vi "单个流程写入.vi"(7 "添加的路径":path, 8 "error in (no error)":errorcluster caption="错误输入（无错误）", 9 "量程":enum16{"低量程", "高量程"}(ring), 10 "测量模式":enum16{"水样测量", "零点核查", "跨度核查", "标样核查", "加标回收"}(ring), 11 "测量参数":enum16{"总磷", "总氮", "氨氮"}(ring)) -> (0 "error out":errorcluster caption="错误输出")   [LabVIEW 2016, in "斯坦道总磷.lvlib"]
panel:
  out "数组 2":u16[][](array[numeric])
  out "大小":i32
  out "交织的数组":u16[](array[numeric]) format="%04x"
  out "数值":i32
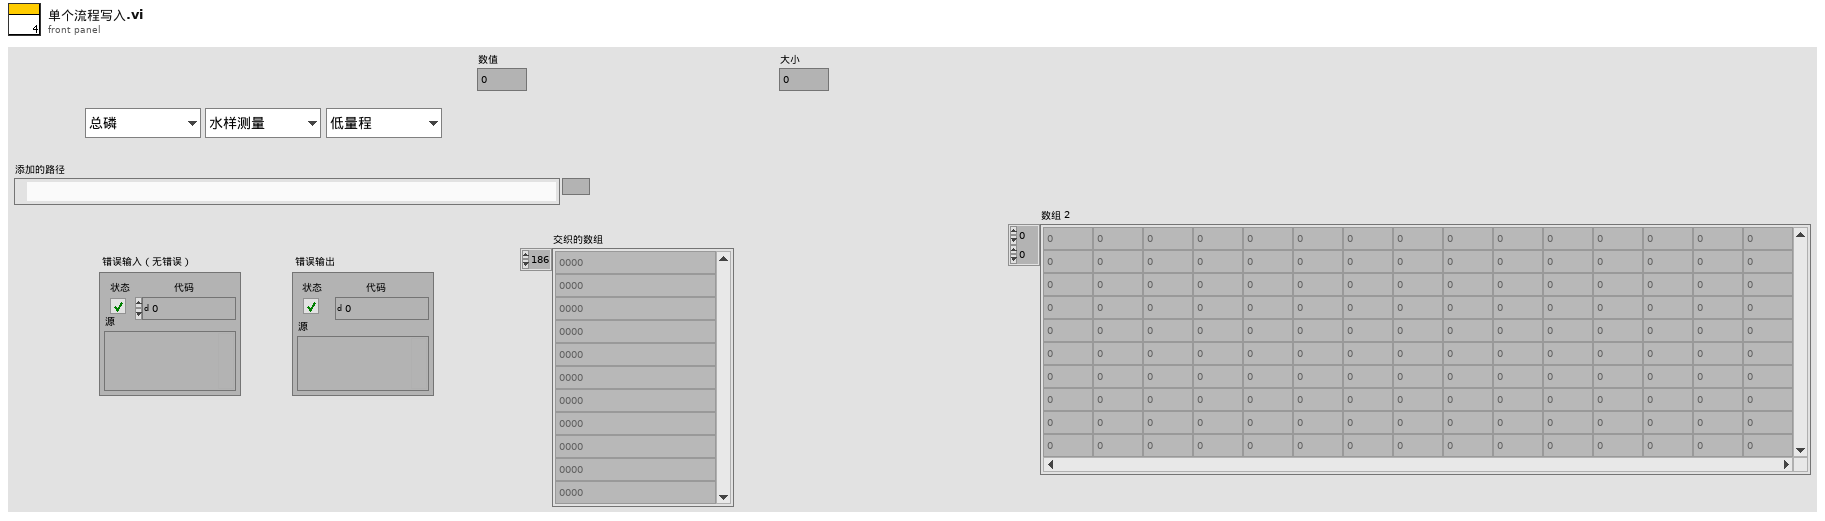
[diagram p1: front panel]
types:
  T1 = cluster{"站号":u16, "starting address":u16, "starting address":u16}
  T2 = cluster{"port":u32, "dac":u8, "adc":u8, "time":u16, "步骤名":string}[]
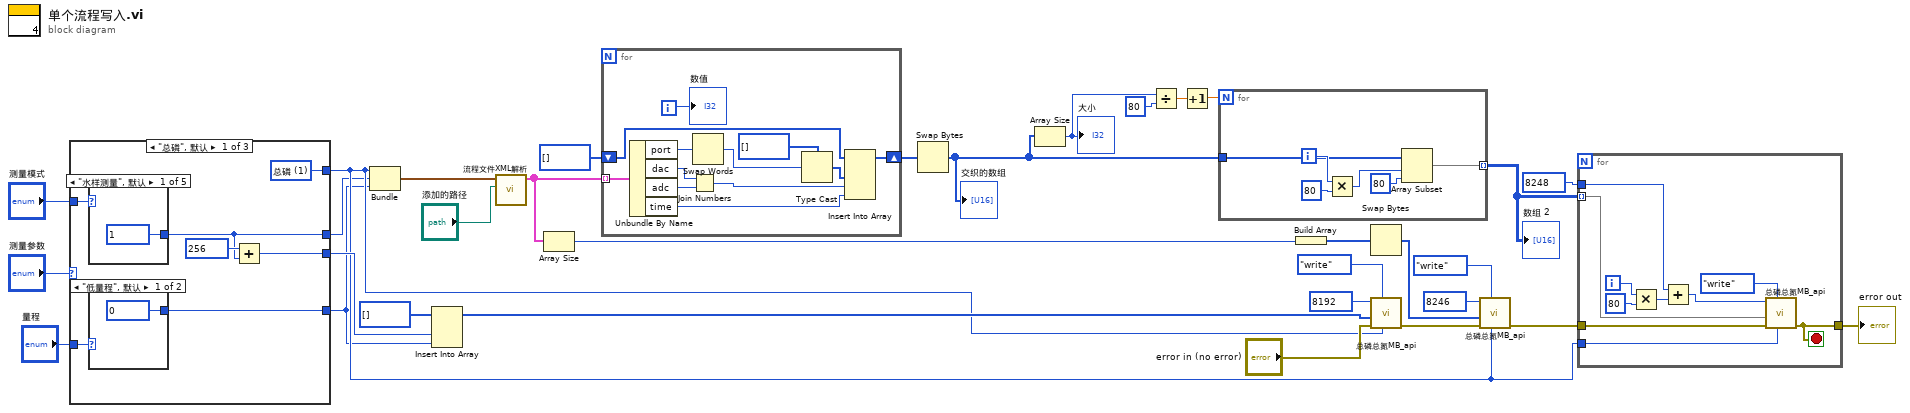
[diagram p0: block diagram]
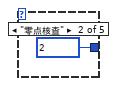
[diagram p2: hidden frame]
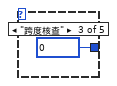
[diagram p3: hidden frame]
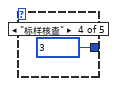
[diagram p4: hidden frame]
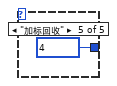
[diagram p5: hidden frame]
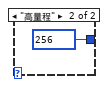
[diagram p6: hidden frame]
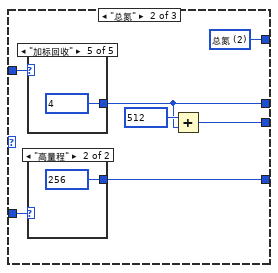
[diagram p7: hidden frame]
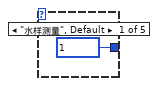
[diagram p8: hidden frame]
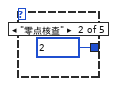
[diagram p9: hidden frame]
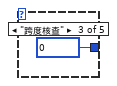
[diagram p10: hidden frame]
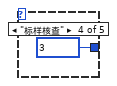
[diagram p11: hidden frame]
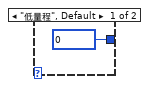
[diagram p12: hidden frame]
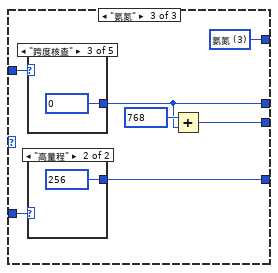
[diagram p13: hidden frame]
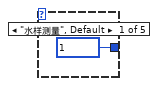
[diagram p14: hidden frame]
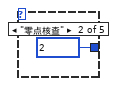
[diagram p15: hidden frame]
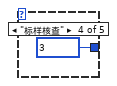
[diagram p16: hidden frame]
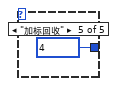
[diagram p17: hidden frame]
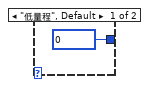
[diagram p18: hidden frame]
diagram:
  n1 = case shown="\"总磷\", 默认" "测量参数" {
    tunnel: "测量模式" -> [w38 w51 w65]
    tunnel: "量程" -> [w39 w52 w66]
    tunnel: [w34 w53 w67] -> w18
    tunnel: [w35 w48 w62] -> w28
    tunnel: [w37 w50 w64] -> w15
    tunnel: [w33 w47 w61] -> w16
    frame "总磷", Default {
      w34 = u16 1 items=["总磷"=1, "总氮"=2, "氨氮"=3] ("站号")
      n2 = case shown="\"水样测量\", 默认" w38 {
        tunnel: [u16 1 ("starting address") u16 2 ("starting address") u16 0 ("starting address") u16 3 ("starting address") u16 4 ("starting address")] -> w33
        frame "水样测量", Default {
        }
        frame "零点核查" {
        }
        frame "跨度核查" {
        }
        frame "标样核查" {
        }
        frame "加标回收" {
        }
      }
      n3 = case shown="\"低量程\", 默认" w39 {
        tunnel: [u16 0 ("starting address") u16 256 ("starting address")] -> w37
        frame "低量程", Default {
        }
        frame "高量程" {
        }
      }
      n4 = Add(x=u16 256 ("starting address"), y=w33) -> (x+y=w35:u16)
    }
    frame "总氮" {
      w53 = u16 2 items=["总磷"=1, "总氮"=2, "氨氮"=3] ("站号")
      n5 = case shown="\"加标回收\"" w51 {
        tunnel: [u16 1 ("starting address") u16 2 ("starting address") u16 0 ("starting address") u16 3 ("starting address") u16 4 ("starting address")] -> w47
        frame "水样测量", Default {
        }
        frame "零点核查" {
        }
        frame "跨度核查" {
        }
        frame "标样核查" {
        }
        frame "加标回收" {
        }
      }
      n6 = case shown="\"高量程\"" w52 {
        tunnel: [u16 0 ("starting address") u16 256 ("starting address")] -> w50
        frame "低量程", Default {
        }
        frame "高量程" {
        }
      }
      n7 = Add(x=u16 512 ("starting address"), y=w47) -> (x+y=w48:u16)
    }
    frame "氨氮" {
      w67 = u16 3 items=["总磷"=1, "总氮"=2, "氨氮"=3] ("站号")
      n8 = case shown="\"跨度核查\"" w65 {
        tunnel: [u16 1 ("starting address") u16 2 ("starting address") u16 0 ("starting address") u16 3 ("starting address") u16 4 ("starting address")] -> w61
        frame "水样测量", Default {
        }
        frame "零点核查" {
        }
        frame "跨度核查" {
        }
        frame "标样核查" {
        }
        frame "加标回收" {
        }
      }
      n9 = case shown="\"高量程\"" w66 {
        tunnel: [u16 0 ("starting address") u16 256 ("starting address")] -> w64
        frame "低量程", Default {
        }
        frame "高量程" {
        }
      }
      n10 = Add(x=u16 768 ("starting address"), y=w61) -> (x+y=w62:u16)
    }
  }
  n11 = Bundle("站号"=w18, "starting address"=w16, "starting address"=w15) -> (w14:T1)  [unwired: 1 in]
  n12 = Insert Into Array(array=u16[] [] ("数组"), new element #1=w28, new element #2=w15) -> (w22:u16[])  [unwired: 1 in]
  n13 = call "流程文件XML解析.vi"("添加的路径"="添加的路径", "参数簇"=w14) -> ("数组"=w6:T2)  [unwired: 9 in]
  n14 = Array Size(array=w6) -> (size(s)=w5:i32)
  n15 = for {
    tunnel: w6 -> [w86] mode=indexing
    shift-right: [w78] -> w11
    shift-left: u16[] [] -> [w76]
    i -> [w85]
    n16 = Unbundle By Name(w86) -> ("port"=w81:u32, "dac"=w84:u8, "adc"=w83:u8, "time"=w79:u16)
    n17 = Join Numbers(hi=w84, lo=w83) -> ((hi.lo)=w80:u16)
    n18 = Swap Words(1:w81) -> (0:w75:u32)
    n19 = Type Cast(type=u16[] [], x=w75) -> (*(type *) &x=w77:u16[])
    n20 = Insert Into Array(array=w76, new element #1=w77, new element #2=w80, new element #3=w79) -> (w78:u16[])  [unwired: 1 in]
    "数值" <- w85
  }
  n21 = Swap Bytes(anything=w11) -> (byte swapped=w8:u16[])
  "交织的数组" <- w8
  n22 = Array Size(array=w8) -> (size(s)=w10:i32)
  "大小" <- w10
  n23 = Divide(x=w10, y=80) -> (x/y=w3:dbl)
  n24 = Increment(x=w3) -> (x+1=w2:dbl)
  n25 = for {
    N: w2 -> [_]
    tunnel: w8 -> [w90]
    tunnel: [w87] -> w7 mode=indexing
    i -> [w92]
    n26 = Multiply(x=w92, y=80) -> (x*y=w89:i32)
    n27 = Array Subset(array=w90, index=w89, length=80 ("y")) -> (w87:u16[])
  }
  "数组 2" <- w7
  n28 = Build Array(w5) -> (w4:i32[])
  n29 = Swap Bytes(anything=w4) -> (byte swapped=w1:i32[])
  n30 = call "总磷总氮MB_api.vi"("Slave ID"=w18, "STEP"=enum16{"open", "read", "write", "close"}."write", "Error in"="error in (no error)", "values"=w22, "starting address"=u16 8192) -> ("error out"=w25:errorcluster)  [unwired: 4 in, 2 out]
  n31 = call "总磷总氮MB_api.vi"("Slave ID"=w18, "STEP"=enum16{"open", "read", "write", "close"}."write", "Error in"=w25, "values"=w1, "starting address"=u16 8246) -> ("error out"=w21:errorcluster)  [unwired: 4 in, 2 out]
  n32 = for {
    tunnel: u16 8248 ("starting address") -> [w96]
    tunnel: w21 -> [w102]
    tunnel: [w100] -> w19
    tunnel: w18 -> [w99]
    tunnel: w7 -> [w98] mode=indexing
    i -> [w95]
    stop <- w100 stop-if-true
    n33 = Multiply(x=w95, y=80) -> (x*y=w94:i32)
    n34 = Add(x=w96, y=w94) -> (x+y=w97:i32)
    n35 = call "总磷总氮MB_api.vi"("Slave ID"=w99, "STEP"=enum16{"open", "read", "write", "close"}."write", "Error in"=w102, "values"=w98, "starting address"=w97) -> ("error out"=w100:errorcluster)  [unwired: 4 in, 2 out]
  }
  "error out" <- w19
